vi "read_database_password.vi"(7 "error_in":errorcluster) -> (0 "error_out":errorcluster, 3 "database_password":string)   [LabVIEW 2020]
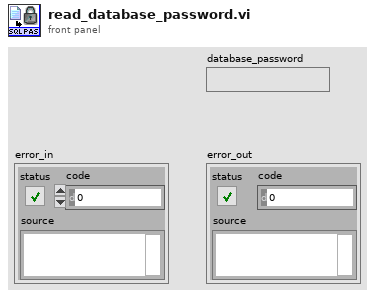
[diagram p1: front panel]
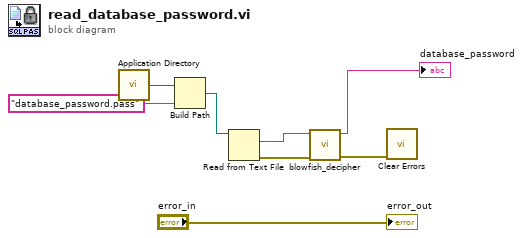
[diagram p0: block diagram]
diagram:
  n1 = call <vilib>:"Application Directory.vi"() -> ("Application Directory"=w8:path)
  n2 = Build Path(base path=w8, name or relative path="database_password.pass") -> (appended path=w6:path)
  n3 = Read from Text File(file (use dialog)=w6) -> (text=w5:string, error out=w3:errorcluster)  [unwired: 3 in, 2 out]
  n4 = call "blowfish_decipher.vi"("error in (no error)"=w3, "Input Text"=w5) -> ("error out"=w2:errorcluster, "data string"=→"database_password":string)  [unwired: 8 in]
  n5 = call <vilib>:"Clear Errors.vi"("error in (no error)"=w2) -> ()  [unwired: 5 in, 2 out]
  "error_out" <- "error_in"
